vi "Get LV Class Default Value By Plug-in Directory.vi"(7 "Use .llb? (F)":bool, 8 "error in (no error)":errorcluster, 9 "options (0x20)":u32=32 format="%.0x", 10 "Plug-in Class Qualified Name":string, 11 "Path To Plug-in Directory":path) -> (0 "error out":errorcluster, 3 "LabVIEW Object out":refnum<class>)   [LabVIEW 2017]
doc: "This VI is a wrapper around both Get LV Class Default Value.vi and Get LV Class Default Value By Name.vi. It is meant to handle the boiler plate code needed to implement a plug-in class architecture.\n\nThis VI can handle classes that have never been saved to disk as well as those that need to be loaded into memory. The <b>Plug-in Class Name</b> can be with or without the file extensions (there may be multiple if the class has one or more containing libraries). If the file extensions are not included, they will be added as lowercase (important on case-sensitive operating systems).\n\nThe <b>Path To Plug-in Directory</b> is used as the base directory from which to load any class not found in memory. If the path is used, it must be a valid absolute path, but the path is only checked if the class is not already in memory. A class named \n \"Y.lvlib:X.lvclass\" \nwill be loaded from \n \"<plug-in directory>\\Y\\X\\X.lvclass\""
uses:
  <vilib>/Utility/error.llb/Error Cluster From Error Code.vi
  <vilib>/ErrorRing/Error Ring.xnode
panel:
  out "Debugging:\nQName":string
  out "Debugging:\nAttempted Class Path":path
  # "These two Debugging indicators may not match the actual qualified name or the actual path of the class even if the class is loaded into memory. It may be that the class at the computed path has a different qualified name than the name requested and that qualified name might already be in memory from another path.  For this reason, if you need these values, it is best to get them from the returned object rather than expose these two values as outputs of this subVI."
  # "The default is to not display the search dialog for missing files since plug-ins might not exist on disk."
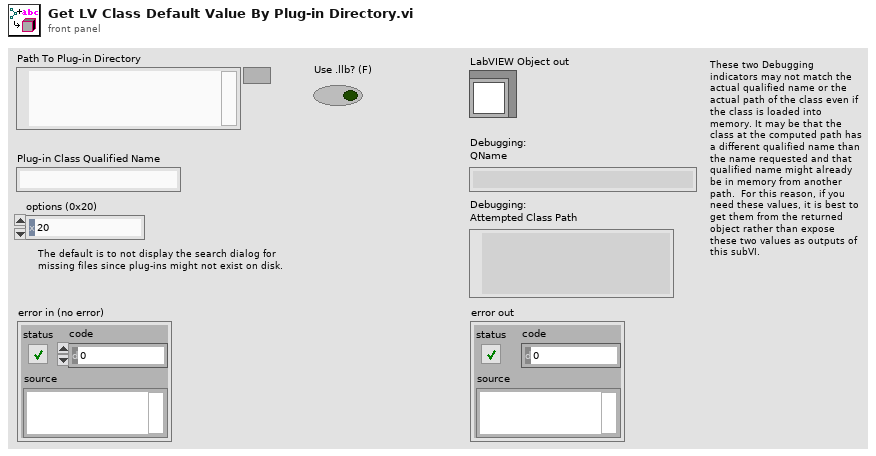
[diagram p1: front panel]
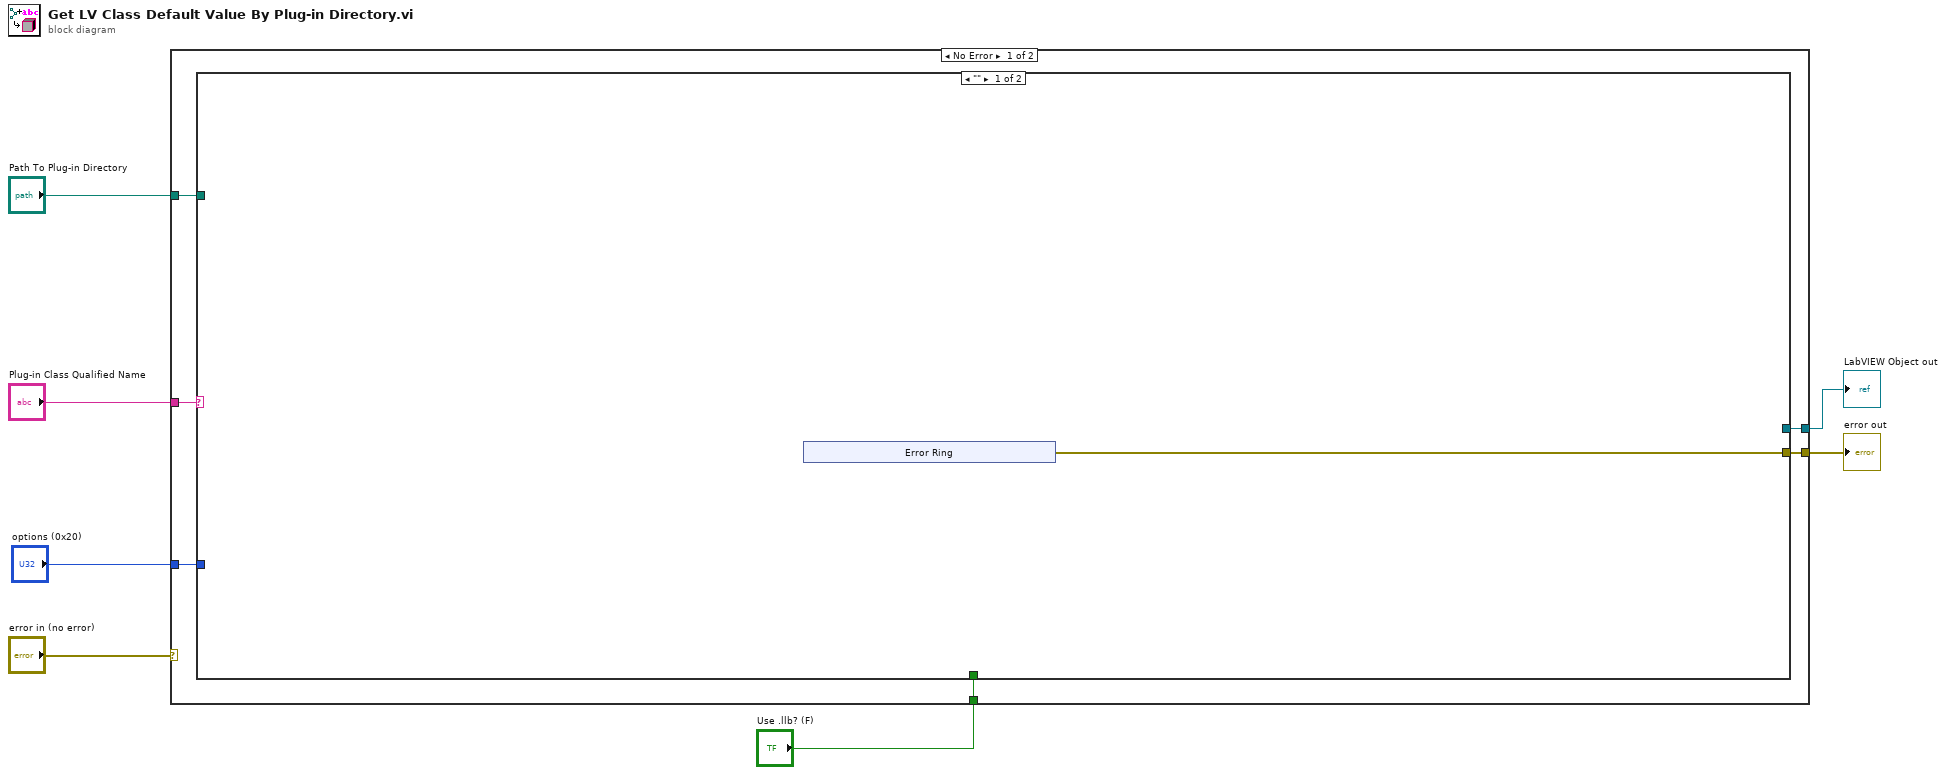
[diagram p0: block diagram]
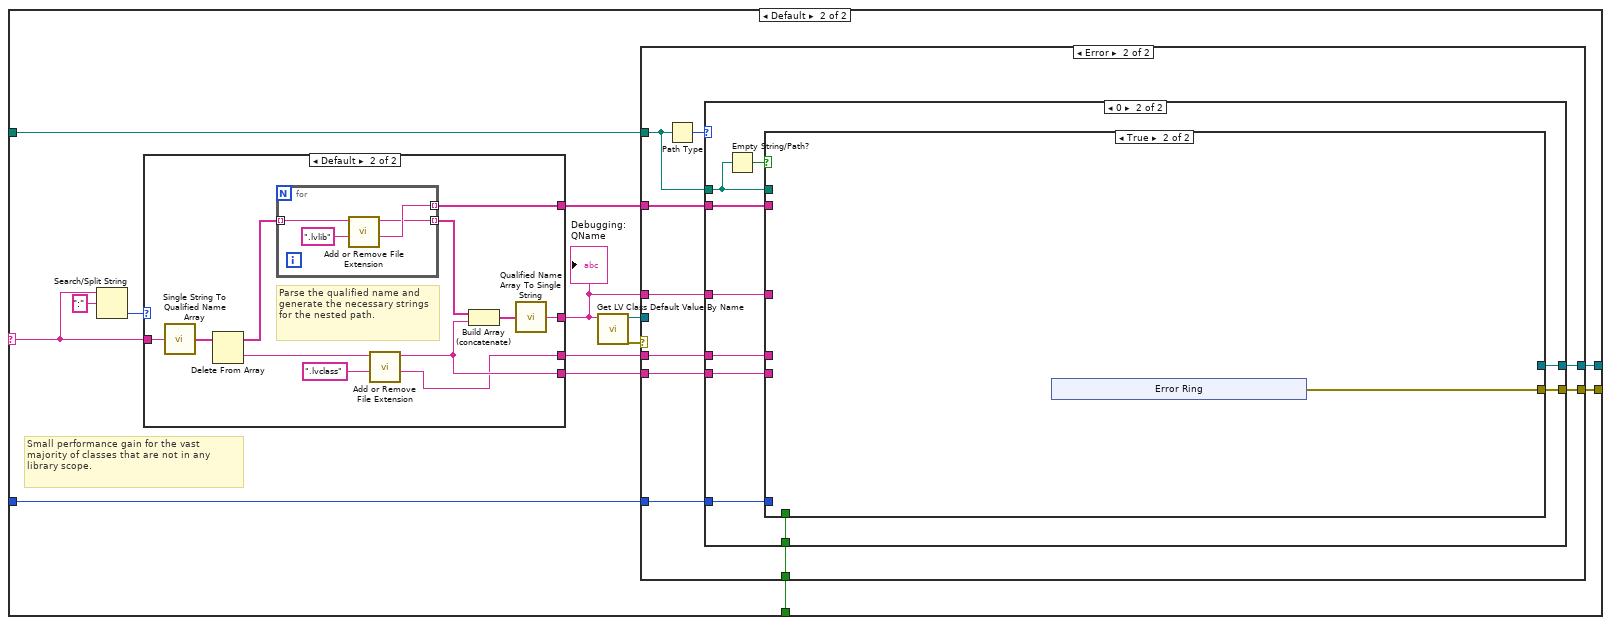
[diagram p2: hidden frame]
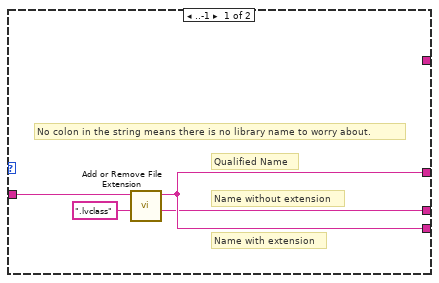
[diagram p3: hidden frame]
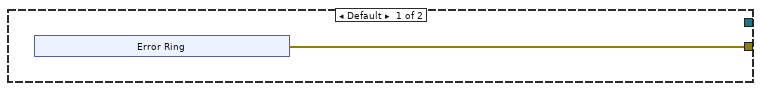
[diagram p5: hidden frame]
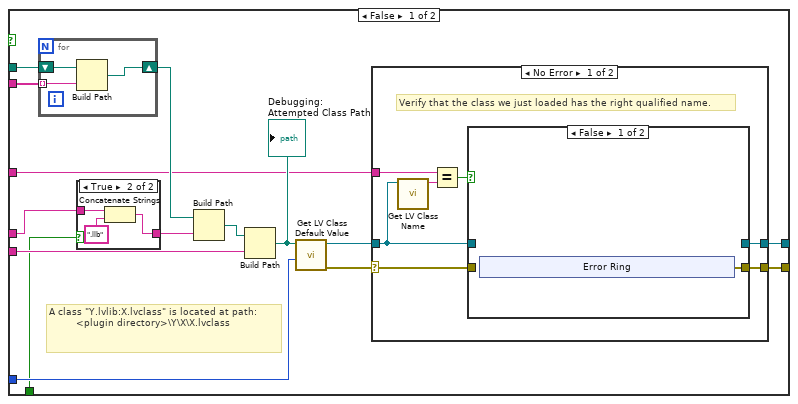
[diagram p6: hidden frame]
diagram:
  n1 = case shown="No Error" "error in (no error)" {
    selector: "error in (no error)" -> [_ w122]
    tunnel: "Plug-in Class Qualified Name" -> [w9 _]
    tunnel: [w13 w122] -> w6
    tunnel: [w12 _] -> w5
    tunnel: "options (0x20)" -> [w11 _]
    tunnel: "Path To Plug-in Directory" -> [w10 _]
    tunnel: "Use .llb? (F)" -> [w8 _]
    frame No Error {
      n2 = case shown="\"\"" w9 {
        selector: w9 -> [_ w23]
        tunnel: [w14 w32] -> w13
        tunnel: [_ w31] -> w12
        tunnel: w11 -> [_ w30]
        tunnel: w10 -> [_ w29]
        tunnel: w8 -> [_ w19]
        frame "" {
          n3 = xnode "Error Ring"() -> ("error out"=w14:errorcluster)
        }
        frame Default {
          # "Small performance gain for the vast majority of classes that are not in any library scope."
          n4 = Search/Split String(string=w23, search string/char (-)=":") -> (offset of match=w21:i32)  [unwired: 1 in, 2 out]
          n5 = case shown="Default" w21 {
            tunnel: [w36 w47] -> w20
            tunnel: [_ w43] -> w26
            tunnel: [w36 w38] -> w25
            tunnel: [w34 w37] -> w24
            tunnel: w23 -> [w35 w44]
            frame ..-1 {
              # "Qualified Name"
              # "Name without extension"
              # "Name with extension"
              # "No colon in the string means there is no library name to worry about."
              n6 = call <vilib>:"Add or Remove File Extension.vi"("File extension with period"=".lvclass" ("search string/char (-)"), "File name with or without extension"=w35) -> ("Without extension"=w34:string, "With extension"=w36:string)  [unwired: 8 in]
            }
            frame Default {
              # "Parse the qualified name and generate the necessary strings for the nested path."
              n7 = call <vilib>:"Single String To Qualified Name Array.vi"("Fully Qualified String"=w44) -> ("Fully Qualified Array"=w42:string[])
              n8 = Delete From Array(array=w42) -> (deleted portion=w40:string, array with subset deleted=w41:string[])  [unwired: 2 in]
              n9 = for {
                tunnel: w41 -> [w51] mode=indexing
                tunnel: [w49] -> w43 mode=indexing
                tunnel: [w48] -> w46 mode=indexing
                n10 = call <vilib>:"Add or Remove File Extension.vi"("File extension with period"=".lvlib" ("search string/char (-)"), "File name with or without extension"=w51) -> ("Without extension"=w49:string, "With extension"=w48:string)  [unwired: 8 in]
              }
              n11 = call <vilib>:"Add or Remove File Extension.vi"("File extension with period"=".lvclass" ("search string/char (-)"), "File name with or without extension"=w40) -> ("Without extension"=w37:string, "With extension"=w38:string)  [unwired: 8 in]
              n12 = Build Array (concatenate)(w46, w38) -> (w45:string[])
              n13 = call <vilib>:"Qualified Name Array To Single String.vi"("Fully Qualified Array"=w45) -> ("Fully Qualified String"=w47:string)
            }
          }
          "Debugging:\nQName" <- w20
          n14 = call <vilib>:"Get LV Class Default Value By Name.vi"("class name"=w20) -> ("error out"=w28:errorcluster, "object"=w27:refnum<class>)  [unwired: 9 in]
          n15 = case shown="Error" w28 {
            selector: w28 -> [w52 _]
            tunnel: [w52 w63] -> w32
            tunnel: [w53 w62] -> w31
            tunnel: w30 -> [_ w61]
            tunnel: w29 -> [_ w60]
            tunnel: w27 -> [w53 _]
            tunnel: w26 -> [_ w58]
            tunnel: w25 -> [_ w57]
            tunnel: w24 -> [_ w56]
            tunnel: w20 -> [_ w55]
            tunnel: w19 -> [_ w54]
            frame No Error {
            }
            frame Error {
              n16 = Path Type(1:w60) -> (0:w59:i16)
              n17 = case shown="0" w59 {
                tunnel: [w64 w78] -> w63
                tunnel: [_ w77] -> w62
                tunnel: w61 -> [_ w76]
                tunnel: w60 -> [_ w75]
                tunnel: w58 -> [_ w73]
                tunnel: w57 -> [_ w72]
                tunnel: w56 -> [_ w71]
                tunnel: w55 -> [_ w70]
                tunnel: w54 -> [_ w69]
                frame Default {
                  n18 = xnode "Error Ring"() -> ("error out"=w64:errorcluster)
                }
                frame 0 {
                  n19 = Empty String/Path?(string/path=w75) -> (empty?=w74:bool)
                  n20 = case shown="True" w74 {
                    tunnel: [w84 w117] -> w78
                    tunnel: [w85 _] -> w77
                    tunnel: w76 -> [w92 _]
                    tunnel: w75 -> [w91 _]
                    tunnel: w73 -> [w86 _]
                    tunnel: w72 -> [w90 _]
                    tunnel: w71 -> [w81 _]
                    tunnel: w70 -> [w82 _]
                    tunnel: w69 -> [w79 _]
                    frame False {
                      # "A class \"Y.lvlib:X.lvclass\" is located at path: \n         <plugin directory>\\Y\\X\\X.lvclass"
                      n21 = for {
                        shift-right: [w115] -> w89
                        shift-left: w91 -> [w116]
                        tunnel: w86 -> [w114] mode=indexing
                        n22 = Build Path(base path=w116, name or relative path=w114) -> (appended path=w115:path)
                      }
                      n23 = case shown="True" w79 {
                        tunnel: w81 -> [w94 w97]
                        tunnel: [w94 w96] -> w80
                        frame False {
                        }
                        frame True {
                          n24 = Concatenate Strings(w97, ".llb" ("Without extension")) -> (w96:string)
                        }
                      }
                      n25 = Build Path(base path=w89, name or relative path=w80) -> (appended path=w88:path)
                      n26 = Build Path(base path=w88, name or relative path=w90) -> (appended path=w93:path)
                      "Debugging:\nAttempted Class Path" <- w93
                      n27 = call <vilib>:"Get LV Class Default Value.vi"("options"=w92, "class path"=w93) -> ("error out"=w83:errorcluster, "object"=w87:refnum<class>)  [unwired: 8 in]
                      n28 = case shown="No Error" w83 {
                        selector: w83 -> [w98 w112]
                        tunnel: w87 -> [w100 w113]
                        tunnel: [w101 w113] -> w85
                        tunnel: [w99 w112] -> w84
                        tunnel: w82 -> [w103 _]
                        frame No Error {
                          # "Verify that the class we just loaded has the right qualified name."
                          n29 = call <vilib>:"Get LV Class Name.vi"("object"=w100) -> ("class name"=w104:string)  [unwired: 9 in, 1 out]
                          n30 = Equal?(x=w103, y=w104) -> (x = y?=w102:bool)
                          n31 = case shown="False" w102 {
                            tunnel: [_ w111] -> w101
                            tunnel: w100 -> [_ w111]
                            tunnel: [w105 w110] -> w99
                            tunnel: w98 -> [_ w110]
                            frame False {
                              n32 = xnode "Error Ring"() -> ("error out"=w105:errorcluster)
                            }
                            frame True {
                            }
                          }
                        }
                        frame Error {
                        }
                      }
                    }
                    frame True {
                      n33 = xnode "Error Ring"() -> ("error out"=w117:errorcluster)
                    }
                  }
                }
              }
            }
          }
        }
      }
    }
    frame Error {
    }
  }
  "error out" <- w6
  "LabVIEW Object out" <- w5
